vi "Dlg Save File.vi"(8 "error in":errorcluster, 11 "CSV in":refnum<class "CSV.lvclass">) -> (0 "error out":errorcluster, 2 "cancelled":bool, 3 "CSV out":refnum<class "CSV.lvclass">)   [LabVIEW 2017, in "Report_lib.lvlib" / "CSV.lvclass"]
doc: "This method call dialog prompt \nwindow for Save existing File"
uses:
  CSV.lvclass
  CSV.lvclass/CSV.ctl
panel:
  out "selected path":path
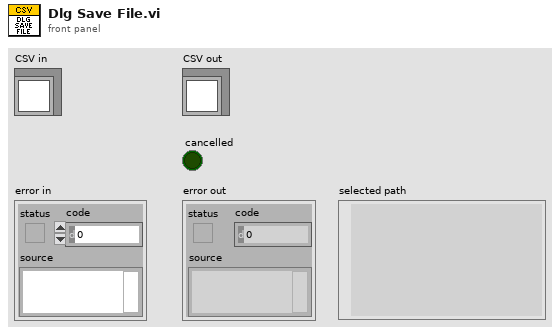
[diagram p1: front panel]
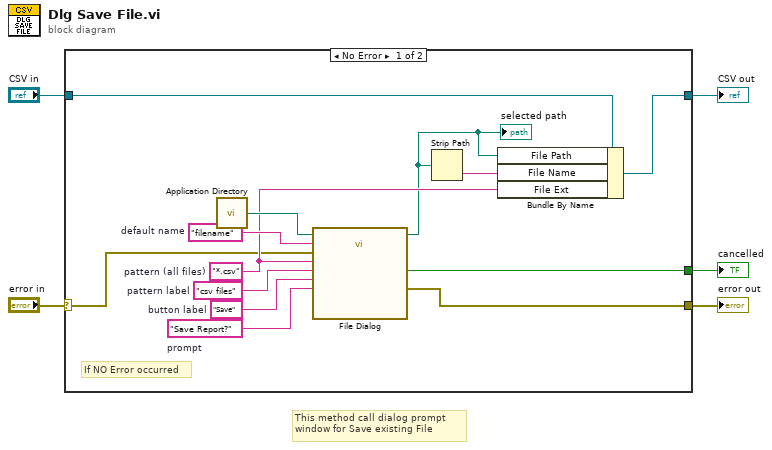
[diagram p0: block diagram]
diagram:
  # "This method call dialog prompt \nwindow for Save existing File"
  n1 = case shown="No Error" "error in" {
    selector: "error in" -> [w7 w20]
    tunnel: [w6 w20] -> w4
    tunnel: [w8 w19] -> w2
    tunnel: "CSV in" -> [w9 w19]
    tunnel: [w10 _] -> w1
    frame No Error {
      w14 = "csv files"  # pattern label
      w15 = "Save Report?"  # prompt
      w16 = "Save"  # button label
      w12 = "*.csv"  # pattern (all files)
      w17 = "filename"  # default name
      # "If NO Error occurred"
      n2 = call <vilib>:"Application Directory.vi"() -> ("Application Directory"=w18:path)
      n3 = call "File Dialog"("start path"=w18, "prompt"=w15, "button label"=w16, "default name"=w17, "error in"=w7, "pattern (all files)"=w12, "pattern label"=w14) -> ("selected path"=w11:path, "cancelled"=w10:bool, "error out"=w6:errorcluster)  [unwired: 5 in, 1 out]
      "selected path" <- w11
      n4 = Strip Path(path=w11) -> (name=w13:string)  [unwired: 1 out]
      n5 = Bundle By Name(cluster=w9, "File Path"=w11, "File Name"=w13, "File Ext"=w12) -> (w8:refnum<class "CSV.lvclass">)
    }
    frame Error {
    }
  }
  "error out" <- w4
  "CSV out" <- w2
  "cancelled" <- w1
